vi "Read Params.vi"(8 "error in (no error)":errorcluster, 11 "Synchronizer in":refnum<class "Synchronizer.lvclass">) -> (0 "error out":errorcluster, 1 "Decimation Factor":u8, 2 "Sequence length":i32=256, 3 "Synchronizer out":refnum<class "Synchronizer.lvclass">)   [LabVIEW 2012, in "Synchronizer.lvclass"]
uses:
  Synchronizer.lvclass
  Synchronizer.lvclass/Synchronizer.ctl
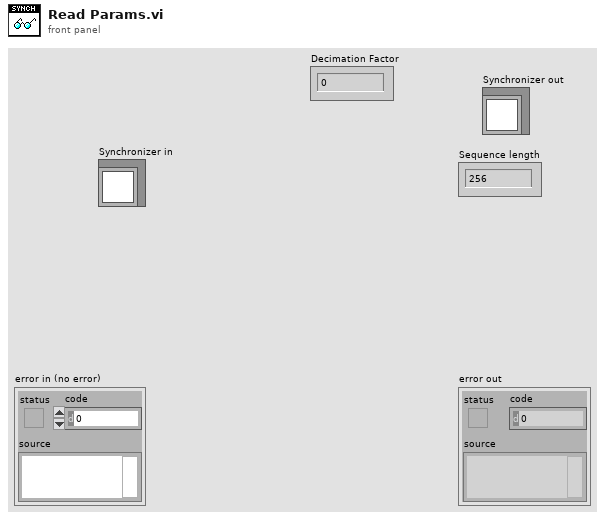
[diagram p1: front panel]
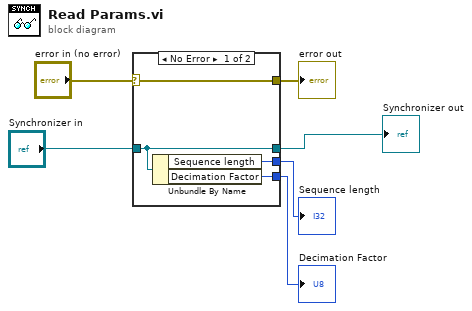
[diagram p0: block diagram]
diagram:
  n1 = case shown="No Error" "error in (no error)" {
    selector: "error in (no error)" -> [w10 w11]
    tunnel: [w10 w11] -> w5
    tunnel: [w9 w12] -> w2
    tunnel: "Synchronizer in" -> [w9 w12]
    tunnel: [w8 _] -> w4
    tunnel: [w7 _] -> w3
    frame No Error {
      n2 = Unbundle By Name(w9) -> ("Sequence length"=w8:i32, "Decimation Factor"=w7:u8)
    }
    frame Error {
    }
  }
  "error out" <- w5
  "Sequence length" <- w4
  "Decimation Factor" <- w3
  "Synchronizer out" <- w2
